vi "Test wrapper.vi"() -> ()   [LabVIEW 2011]
uses:
  <vilib>/Analysis/2dsp.llb/2D Complex FFT.vi
  <vilib>/Analysis/NI_AALPro.lvlib
panel:
  in  "DCborderWidth":i32=64
  out "return 2":i32
  out "CUDA Return":i32
  out "return":i32
  out "e":dbl=1.0
  out "u":dbl
  in  "e_desired":sgl=1.0
  in  "Save\nAmplitudes":bool=TRUE
  in  "deviceId":i32
  in  "Intensity":sgl[](array[numeric])=[1.0, 1.0, 1.0, 1.0, 1.0, 1.0, 1.0, 1.0, 1.0]
  in  "Polynomial Coefficients":sgl[](array[numeric])=[128.0, 0.0, 0.0, 40.0, 0.0, 0.0, 0.0, 0.0, 0.0, 0.0, 0.0, 0.0, 0.0, 0.0, 0.0, 0.0, 0.0, 0.0, 0.0, 0.0, 0.0, 0.0, 0.0, 0.0, 0.0, 0.0, 0.0, 0.0, 0.0, 0.0, 0.0, 0.0, 0.0, 0.0, 0.0, 0.0, 0.0, 0.0, 0.0, 0.0, 0.0, 0.0, 0.0, 0.0, 0.0, 0.0, 0.0, 0.0, 0.0, 0.0, 0.0, 0.0, 0.0, 0.0, 0.0, 0.0, 0.0, 0.0, 0.0, 0.0, 0.0, 0.0, 0.0, 0.0, 0.0, 0.0, 0.0, 0.0, 0.0, 0.0, 0.0, 0.0, 0.0, 0.0, 0.0, 0.0, 0.0, 0.0, 0.0, 0.0, 0.0, 0.0, 0.0, 0.0, 0.0, 0.0, 0.0, 0.0, 0.0, 0.0, 0.0, 0.0, 0.0, 0.0, 0.0, 0.0, 0.0, 0.0, 0.0, 0.0, 0.0, 0.0, 0.0, 0.0, 0.0, 0.0, 0.0, 0.0, 0.0, 0.0, 0.0, 0.0, 0.0, 0.0, 0.0, 0.0, 0.0, 0.0, 0.0, 0.0]
  in  "alpha RPC":sgl=1.0
  in  "Polynomial Order":i32=3 min=3 max=7 step=1
  in  "Use polynomial LUT":bool
  out "error out":errorcluster
  in  "Aberration Correction On":bool
  in  "Aberration Correction":sgl[](array[numeric])=array[262144 elements]
  in  "TrueFrame":i32=3
  in  "Number of \ntime to execute":i32=1
  out "Average \nexecution time":dbl=3.1616161616161618
  in  "GO":bool
  in  "stop program":bool
  out "Amplitudes/weights":sgl[][](graph)=[[nan, nan, nan, nan, nan, nan, nan, nan, nan, nan], [nan, nan, nan, nan, nan, nan, nan, nan, nan, nan], [nan, nan, nan, nan, nan, nan, nan, nan, nan, nan], [nan, nan, nan, nan, nan, nan, nan, nan, nan, nan], [nan, nan, nan, nan, nan, nan, nan, nan, nan, nan], [nan, nan, nan, nan, nan, nan, nan, nan, nan, nan], [nan, nan, nan, nan, nan, nan, nan, nan, nan, nan], [nan, nan, nan, nan, nan, nan, nan, nan, nan, nan], [nan, nan, nan, nan, nan, nan, nan, nan, nan, nan]]
  out "Calculated image plane":dbl[][](graph)
  out "Generated Hologram":u8[][](graph)
  in  "method":i32(ring)=2 items=["Lenses and Gratings (3D)", "Gerchberg-Saxton (3D)", "Gerchberg-Saxton FFT (2D)"]
  in  "z":sgl[](array[numeric])=[0.0, 0.0, 0.0, 0.0, 0.0, 0.0, 0.0, 0.0, 0.0]
  in  "y":sgl[](array[numeric])=[40.0, 40.0, -40.0, -40.0, 0.0, 0.0, 40.0, -40.0, 0.0]
  in  "x":sgl[](array[numeric])=[40.0, -40.0, 40.0, -40.0, 40.0, -40.0, 0.0, 0.0, 0.0]
  in  "N_iterations":i32=10
  in  "SLM enabled":bool
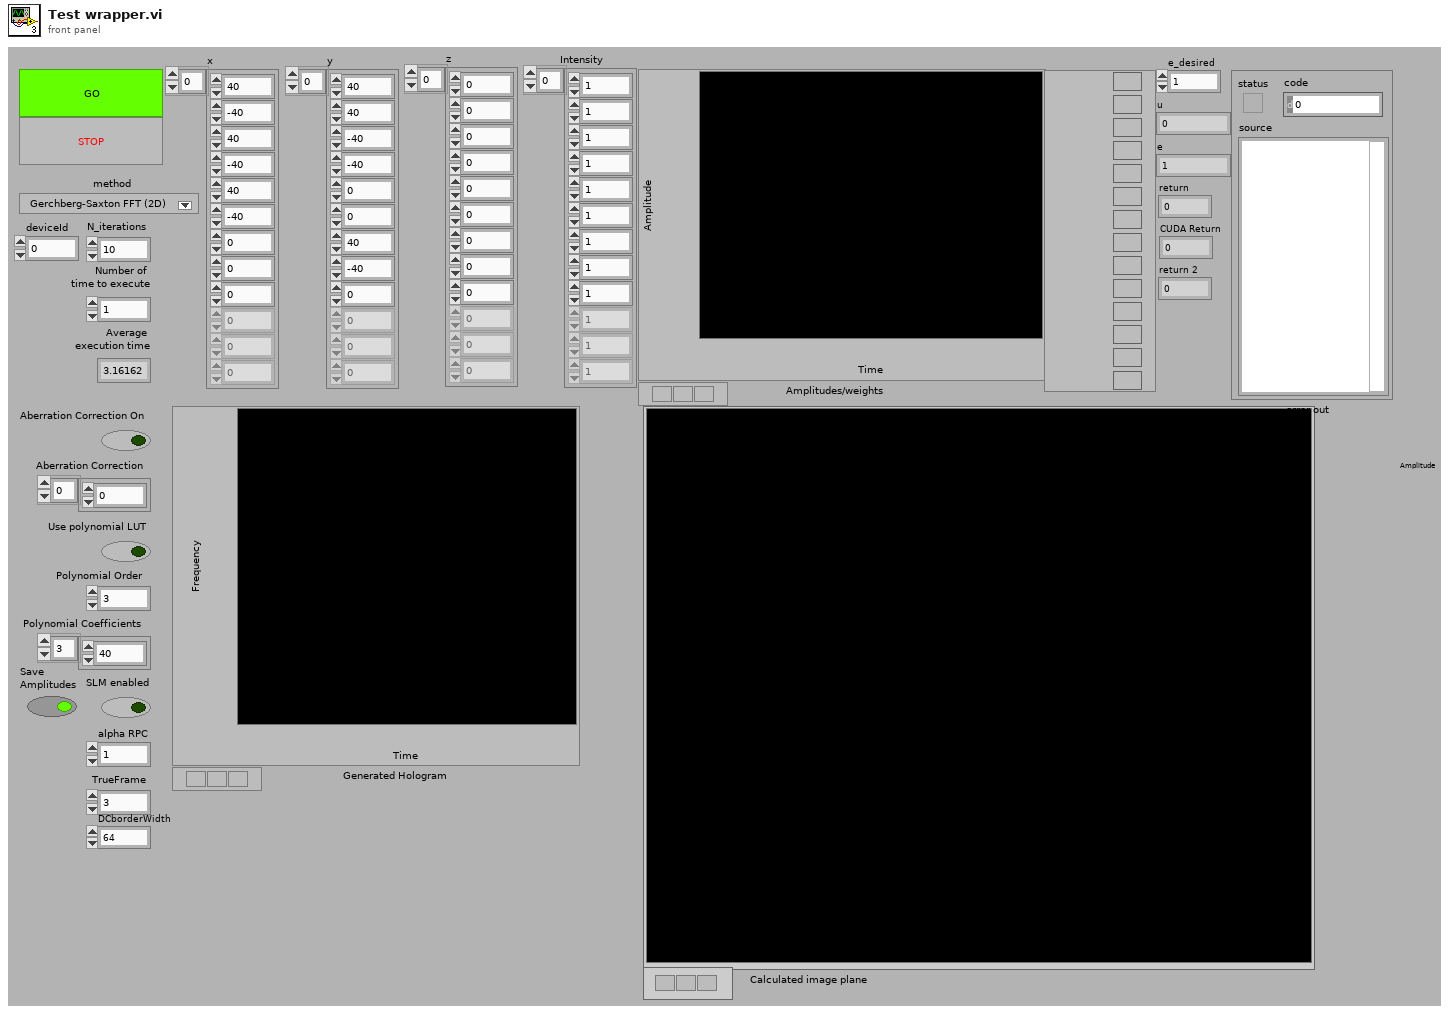
[diagram p1: front panel]
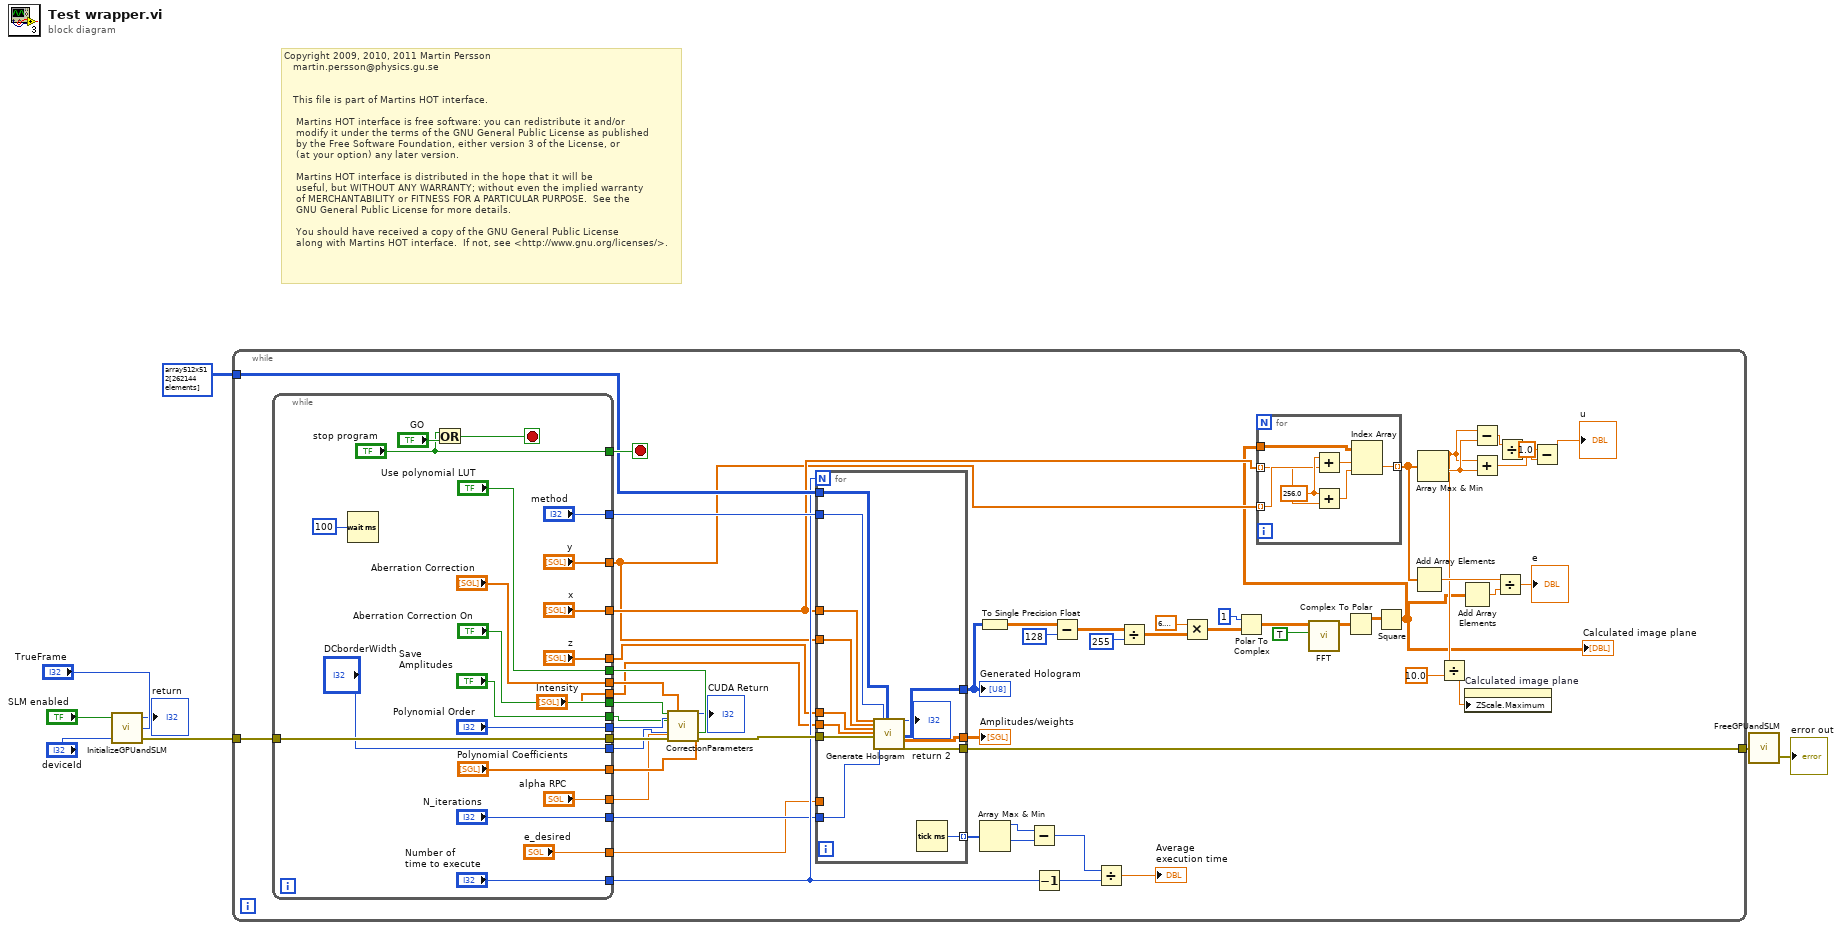
[diagram p0: block diagram]
diagram:
  # "Copyright 2009, 2010, 2011 Martin Persson \n   martin.persson@physics.gu.se\n\n\n   This file is part of Martins HOT interface.\n\n    Martins HOT interface is free software: you can redistribute it and/or \n    modify it under the terms of the GNU General Public License as published \n    by the Free Software Foundation, either version 3 of the License, or\n    (at your option) any later version.\n\n    Martins HOT interface is distributed in the hope that it will be \n    useful, but WITHOUT ANY WARRANTY; without even the implied warranty\n    of MERCHANTABILITY or FITNESS FOR A PARTICULAR PURPOSE.  See the\n    GNU General Public License for more details.\n\n    You should have received a copy of the GNU General Public License\n    along with Martins HOT interface.  If not, see <http://www.gnu.org/licenses/>."
  n1 = call "InitializeGPUandSLM.vi"("TrueFrame"="TrueFrame", "deviceId"="deviceId", "SLM enabled"="SLM enabled") -> ("CUDA/SLM error"=w2:errorcluster, "return"=→"return":i32)  [unwired: 1 in]
  n2 = while {
    tunnel: w2 -> [w43]
    tunnel: [w63] -> w7
    tunnel: u8[][] array512x512[262144 elements] ("Default") -> [w51]
    stop <- w64 stop-if-true
    n3 = while {
      tunnel: ["stop program"] -> w64
      tunnel: w43 -> [w102]
      tunnel: [w102] -> w42
      tunnel: ["alpha RPC"] -> w29
      tunnel: ["Use polynomial LUT"] -> w40
      tunnel: ["Aberration Correction On"] -> w39
      tunnel: ["method"] -> w38
      tunnel: ["Number of \ntime to execute"] -> w37
      tunnel: ["y"] -> w26
      tunnel: ["z"] -> w36
      tunnel: ["x"] -> w27
      tunnel: ["Polynomial Order"] -> w35
      tunnel: ["Aberration Correction"] -> w34
      tunnel: ["Polynomial Coefficients"] -> w33
      tunnel: ["N_iterations"] -> w32
      tunnel: ["Intensity"] -> w31
      tunnel: ["Save\nAmplitudes"] -> w30
      tunnel: ["e_desired"] -> w28
      tunnel: ["DCborderWidth"] -> w9
      stop <- w104 stop-if-true
      n4 = Wait (ms)(milliseconds to wait=u32 100) -> ()  [unwired: 1 out]
      n5 = Or(x="stop program", y="GO") -> (x .or. y?=w104:bool)
    }
    n6 = call "CorrectionParameters.vi"("Aberration Correction On"=w39, "Aberration Correction"=w34, "Polynomial Order"=w35, "SaveAmplitudes"=w30, "Polynomial Coefficients"=w33, "DCborderWidth"=w9, "Use polynomial LUT"=w40, "error in"=w42, "AlphaRPC"=w29) -> ("CUDA Return"=→"CUDA Return":i32, "error out"=w44:errorcluster)  [unwired: 5 in]
    n7 = for {
      N: w37 -> [_]
      tunnel: w44 -> [w85]
      tunnel: w32 -> [w84]
      tunnel: w26 -> [w83]
      tunnel: w36 -> [w82]
      tunnel: w38 -> [w81]
      tunnel: [w80] -> w65
      tunnel: [w79] -> w63
      tunnel: [w78] -> w52
      tunnel: w51 -> [w77]
      tunnel: w27 -> [w76]
      tunnel: w31 -> [w75]
      tunnel: [w74] -> w50 mode=indexing
      tunnel: w28 -> [_]
      n8 = call "Generate Hologram.vi"("x"=w76, "y"=w83, "z"=w82, "spot_intensities"=w75, "CUDA/SLM error in"=w85, "N_iterations"=w84, "method"=w81, "CGH in"=w77) -> ("return"=→"return 2":i32, "CGH out"=w78:u8[][], "weights"=w80:sgl[][], "CUDA/SLM error out"=w79:errorcluster)  [unwired: 16 in]
      n9 = Tick Count (ms)() -> (millisecond timer value=w74:u32)
    }
    "Generated Hologram" <- w52
    "Amplitudes/weights" <- w65
    n10 = To Single Precision Float(number=w52) -> (single precision float=w58:sgl[][])
    n11 = Array Max & Min(array=w50) -> (max value=w49:u32, min value=w48:u32)  [unwired: 2 out]
    n12 = Subtract(x=w49, y=w48) -> (x-y=w47:u32)
    n13 = Decrement(x=w37) -> (x-1=w41:i32)
    n14 = Subtract(x=w58, y=128) -> (x-y=w57:sgl[][])
    n15 = Divide(x=w47, y=w41) -> (x/y=→"Average \nexecution time":dbl)
    n16 = Divide(x=w57, y=255) -> (x/y=w60:sgl[][])
    n17 = Multiply(x=6.283185307179586, y=w60) -> (x*y=w54:dbl[][])
    n18 = Polar To Complex(1:w54, 2:1) -> (0:w53:cdb[][])
    n19 = call-poly <vilib>:"FFT.vi"("shift?"=TRUE, "X"=w53) -> ("FFT {X}"=w56:cdb[][])  [unwired: 2 in, 7 out]
    n20 = Complex To Polar(r * e^(i*theta)=w56) -> (r=w15:dbl[][])  [unwired: 1 out]
    n21 = Square(x=w15) -> (x^2=w11:dbl[][])
    "Calculated image plane" <- w11
    n22 = for {
      tunnel: w11 -> [w72]
      tunnel: w27 -> [w66] mode=indexing
      tunnel: w26 -> [w67] mode=indexing
      tunnel: [w68] -> w21 mode=indexing
      w70 = sgl 256.0 ("x")
      n23 = Add(x=w70, y=w67) -> (x+y=w71:sgl)
      n24 = Add(x=w70, y=w66) -> (x+y=w69:sgl)
      n25 = Index Array(array=w72, index (row)=w71, index (col)=w69) -> (element=w68:dbl)
    }
    n26 = Add Array Elements(numeric array=w21) -> (sum=w20:dbl)
    n27 = Array Max & Min(array=w21) -> (max value=w14:dbl, min value=w24:dbl)  [unwired: 2 out]
    n28 = Divide(x=w14, y=10.0) -> (x/y=w13:dbl)
    n29 = Add Array Elements(numeric array=w11) -> (sum=w22:dbl)
    n30 = property on="Calculated image plane" class="IntGraph (strict)"("ZScale.Maximum"=w13) -> ()  [unwired: 2 in, 2 out]
    n31 = Subtract(x=w14, y=w24) -> (x-y=w25:dbl)
    n32 = Add(x=w14, y=w24) -> (x+y=w23:dbl)
    n33 = Divide(x=w20, y=w22) -> (x/y=→"e":dbl)
    n34 = Divide(x=w25, y=w23) -> (x/y=w17:dbl)
    n35 = Subtract(x=1.0, y=w17) -> (x-y=→"u":dbl)
  }
  n36 = call "FreeGPUandSLM.vi"("error in"=w7) -> ("error out"=→"error out":errorcluster)  [unwired: 1 out]
